vi "Wait.vi"(8 "error in (no error)":errorcluster, 10 "Time to Wait (ms)":u32, 11 "VISA Refnum in":refnum<visa-resource-name>) -> (0 "error out":errorcluster, 3 "VISA Refnum out":refnum<visa-resource-name>)   [LabVIEW 2017, in "SmartMotor.lvclass"]
uses:
  SmartMotor.lvclass
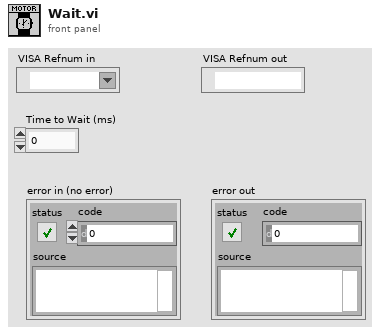
[diagram p1: front panel]
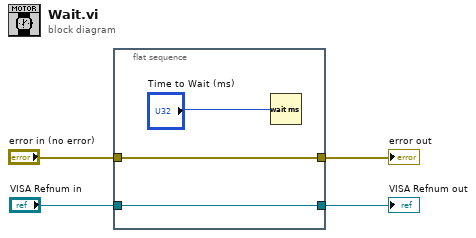
[diagram p0: block diagram]
diagram:
  n1 = flat-sequence {
    tunnel: "VISA Refnum in" -> [w7]
    tunnel: "error in (no error)" -> [w6]
    tunnel: [w7] -> w3
    tunnel: [w6] -> w4
    frame #0 {
      n2 = Wait (ms)(milliseconds to wait="Time to Wait (ms)") -> ()  [unwired: 1 out]
    }
  }
  "error out" <- w4
  "VISA Refnum out" <- w3
